vi "ResolveURLbyUsingInfoCode.vi"(7 "Type":T1=".zip", 8 "error in (no error)":errorcluster, 11 "infocode":string) -> (0 "error out":errorcluster={"status"=TRUE, "code"=7, "source"="ResolveURLbyUsingInfoCode.vi<ERR>\nhttp://digital.ni.com/express.nsf/bycode/exvefe\n\n\n<b>Complete call chain:</b>\r\n     ResolveURLbyUsingInfoCode.vi"}, 1 "whole match":string, 2 "Folder and file":string, 3 "Server name":string, 4 "Infocode URL":string)   [LabVIEW 2020]
uses:
  <vilib>/regexp/Match Regular Expression.xnode
  Controls/DownloadFileType.ctl
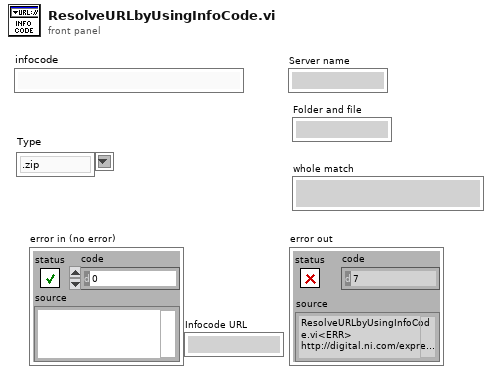
[diagram p1: front panel]
types:
  T1 = typedef "DownloadFileType.ctl" = string
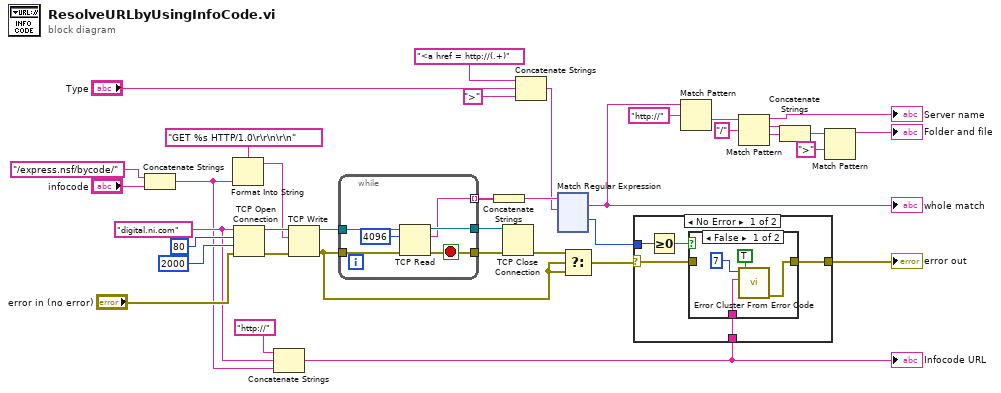
[diagram p0: block diagram]
diagram:
  w14 = "digital.ni.com" ("address")
  n1 = Concatenate Strings("/express.nsf/bycode/" ("address"), "infocode") -> (w13:string)
  n2 = Format Into String(format string="GET %s HTTP/1.0\r\r\n\r\n" ("HTTP Header"), w13) -> (resulting string=w25:string)  [unwired: 2 in, 1 out]
  n3 = TCP Open Connection(address=w14, remote port or service name=u16 80 ("local port"), timeout ms (60000)=2000, error in (no error)="error in (no error)") -> (connection ID=w35:refnum<k5>, error out=w36:errorcluster)  [unwired: 1 out]
  n4 = Concatenate Strings("http://" ("string"), w14, w13) -> (w12:string)
  "Infocode URL" <- w12
  n5 = TCP Write(connection ID=w35, data in=w25, error in (no error)=w36) -> (connection ID out=w34:refnum<k5>, error out=w28:errorcluster)  [unwired: 2 out]
  n6 = while {
    tunnel: w28 -> [w43]
    tunnel: w34 -> [w42]
    tunnel: [w40] -> w33
    tunnel: [w39] -> w32
    tunnel: [w38] -> w30 mode=indexing
    stop <- w39 stop-if-true
    n7 = TCP Read(connection ID=w42, bytes to read=4096, error in (no error)=w43) -> (connection ID out=w40:refnum<k5>, data out=w38:string, error out=w39:errorcluster)  [unwired: 2 out]
  }
  n8 = Concatenate Strings(w30) -> (w22:string)
  n9 = TCP Close Connection(connection ID=w33, error in (no error)=w32) -> (error out=w29:errorcluster)  [unwired: 2 out]
  n10 = Concatenate Strings("<a href = http://(.+)" ("regular expression"), "Type", ">" ("regular expression")) -> (w19:string)
  n11 = xnode "Match Regular Expression"("input string"=w22, "regular expression"=w19) -> ("whole match"=w11:string, "offset past match"=w17:i32)  [unwired: 4 in, 3 out]
  "whole match" <- w11
  n12 = Select(t=w29, s=w28, f=w28) -> (s? t:f=w18:errorcluster)
  n13 = case shown="No Error" w18 {
    selector: w18 -> [w46 w54]
    tunnel: w17 -> [w48 _]
    tunnel: [w45 w54] -> w16
    tunnel: w12 -> [w44 _]
    frame No Error {
      n14 = Greater Or Equal To 0?(x=w48) -> (x >= 0?=w47:bool)
      n15 = case shown="False" w47 {
        tunnel: w46 -> [_ w53]
        tunnel: [w50 w53] -> w45
        tunnel: w44 -> [w49 _]
        frame False {
          n16 = call <vilib>:"Error Cluster From Error Code.vi"("show call chain? (False)"=TRUE, "error message (\"\")"=w49, "error code (0)"=7) -> ("error out"=w50:errorcluster)  [unwired: 6 in]
        }
        frame True {
        }
      }
    }
    frame Error {
    }
  }
  "error out" <- w16
  n17 = Match Pattern(string=w11, regular expression="http://") -> (after substring=w9:string)  [unwired: 1 in, 3 out]
  n18 = Match Pattern(string=w9, regular expression="/") -> (before substring=→"Server name":string, match substring=w6:string, after substring=w5:string)  [unwired: 1 in, 1 out]
  n19 = Concatenate Strings(w6, w5) -> (w3:string)
  n20 = Match Pattern(string=w3, regular expression=">") -> (before substring=→"Folder and file":string)  [unwired: 1 in, 3 out]
